vi "daq_laser_sensors.vi"() -> ()   [LabVIEW 2018]
uses:
  validated_u32.ctl
  <vilib>/rvi/eio/common/nirviEmuTemplateMethod_errors.vi
  <vilib>/rvi/Emulation/niFpgaEmulationIsFPGAContextNoSignature.vi
  <vilib>/rvi/DataTransferAndStorage/Container/Common/niFpgaContainerGetUniqueNameForEmu.vi
  <vilib>/rvi/Memory/Memory_Emulation/niFpgaMemoryEmulationCacheClearOnFirstRun.vi
  <vilib>/rvi/Memory/Memory_Emulation/nirvimemoryEmulationManagerCache_MakeExclusive.vi
  <vilib>/rvi/Memory/Memory_Emulation/niFpgaMemoryEmulationValidateCache.vi
  <vilib>/rvi/Memory/Memory_Emulation/nirvimemoryEmulationManagerCache_InsertValue.vi
  <vilib>/Utility/error.llb/Clear Errors.vi
  <vilib>/rvi/Memory/Memory_Emulation/nirvimemoryEmulationManagerCache_ReleaseExclusive.vi
  <vilib>/rvi/Memory/Memory_Emulation/nirvimemoryEmulationManagerCache_GetValue.vi
  <vilib>/rvi/Memory/Memory_Emulation/nirvimemoryEmulationManagerCache_SetValue.vi
  <vilib>/rvi/Emulation/niFpgaProcessEmulError.vi
  <vilib>/rvi/Emulation/niFpgaSctlEmulationGetInTimedLoop.vi
  <vilib>/eio/EIONode/EIONode.xnode
  <vilib>/rvi/DataTransferAndStorage/Container/XNode/niFpgaContainer.xnode
  <vilib>/rvi/DataTransferAndStorage/Register/Emulation/niFpgaRegisterEmulation.vi
panel:
  in  "timestamp":u32
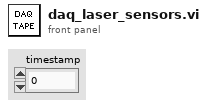
[diagram p1: front panel]
types:
  T1 = typedef "validated_u32.ctl" = cluster{"valid":bool, "value":u32}
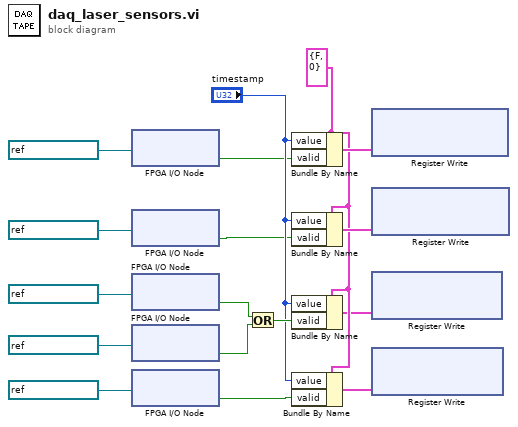
[diagram p0: block diagram]
diagram:
  w12 = T1 {"valid"=FALSE, "value"=0} ("Cluster")
  n1 = xnode "FPGA I/O Node"("FPGA I/O In"=refnum<k21> "Mod2/DIO1") -> ("I/O Item"=w2:bool)  [unwired: 1 out]
  n2 = xnode "FPGA I/O Node"("FPGA I/O In"=refnum<k21> "Mod2/DIO2") -> ("I/O Item"=w1:bool)  [unwired: 1 out]
  n3 = xnode "FPGA I/O Node"("FPGA I/O In"=refnum<k21> "Mod2/DIO3") -> ("I/O Item"=w8:bool)  [unwired: 1 out]
  n4 = xnode "FPGA I/O Node"("FPGA I/O In"=refnum<k21> "Mod2/DIO4") -> ("I/O Item"=w7:bool)  [unwired: 1 out]
  n5 = xnode "FPGA I/O Node"("FPGA I/O In"=refnum<k21> "Mod2/DIO5") -> ("I/O Item"=w6:bool)  [unwired: 1 out]
  n6 = Or(x=w8, y=w7) -> (x .or. y?=w9:bool)
  n7 = Bundle By Name(cluster=w12, "value"="timestamp", "valid"=w2) -> (w14:T1)
  n8 = Bundle By Name(cluster=w12, "value"="timestamp", "valid"=w1) -> (w13:T1)
  n9 = Bundle By Name(cluster=w12, "value"="timestamp", "valid"=w9) -> (w11:T1)
  n10 = Bundle By Name(cluster=w12, "value"="timestamp", "valid"=w6) -> (w10:T1)
  n11 = xnode "Register Write"("Data"=w14) -> ()  [unwired: 1 in, 1 out]
  n12 = xnode "Register Write"("Data"=w13) -> ()  [unwired: 1 in, 1 out]
  n13 = xnode "Register Write"("Data"=w11) -> ()  [unwired: 1 in, 1 out]
  n14 = xnode "Register Write"("Data"=w10) -> ()  [unwired: 1 in, 1 out]
